vi "Test_NoData_NoneFound.vi"(8 "error in (no error)":errorcluster, 11 "TestCase in":refnum<class "TestCurrentValueTable.lvclass">) -> (0 "error out":errorcluster, 3 "TestCase out":refnum<class "TestCurrentValueTable.lvclass">)   [LabVIEW 2015, in "TestCurrentValueTable.lvclass"]
uses:
  TestCurrentValueTable.lvclass
  <vilib>/addons/_JKI Toolkits/VI Tester/TestCase.llb/TestCase.lvclass
  CurrentValueTable.lvclass
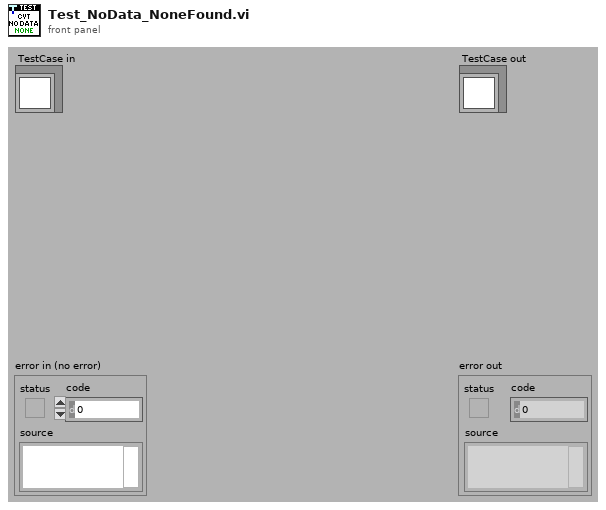
[diagram p1: front panel]
types:
  T1 = typedef "CurrentValueTable.lvlib/CurrentValueTable.lvclass/CurrentValueTable Reference.ctl" = refnum<data-value>
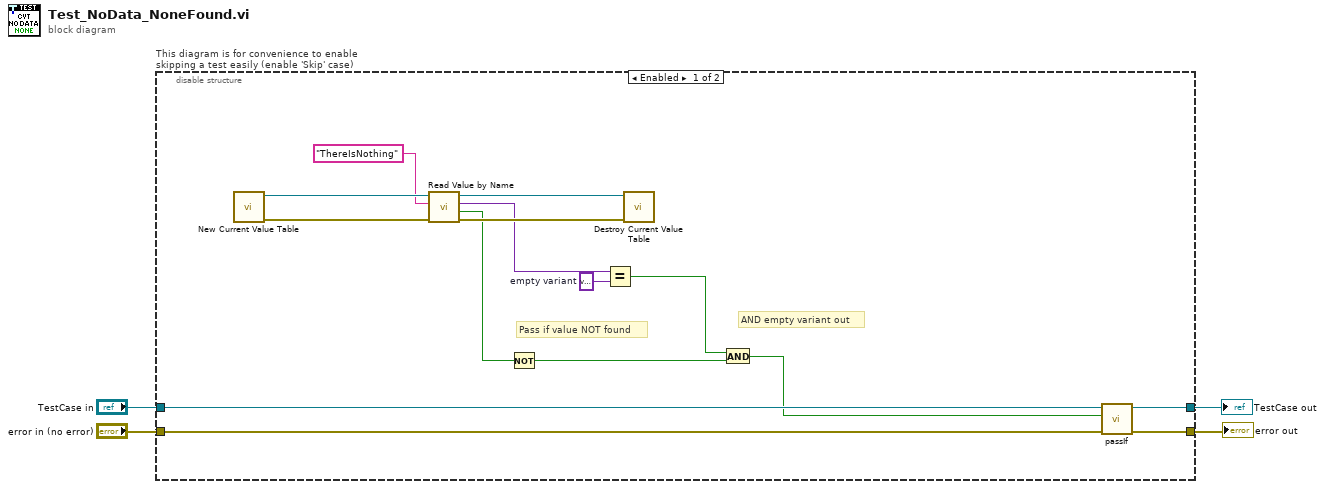
[diagram p0: block diagram]
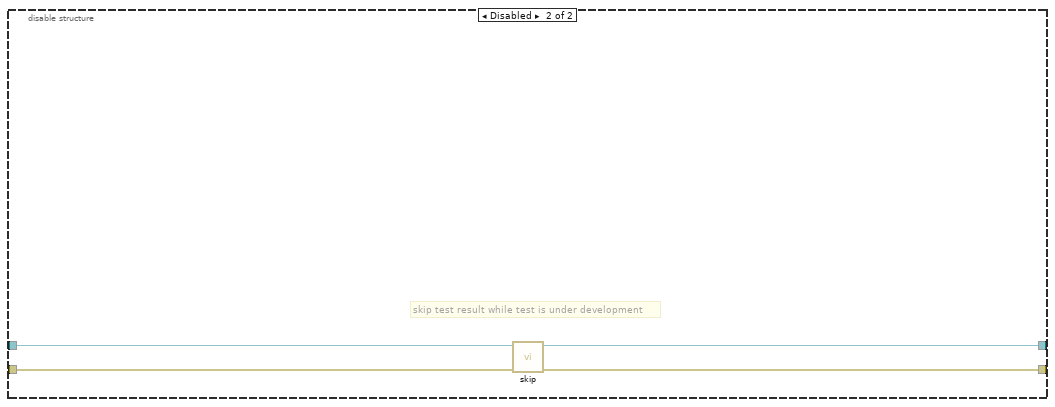
[diagram p2: hidden frame]
diagram:
  n1 = disable-structure "This diagram is for convenience to enable skipping a test easily (enable 'Skip' case)" shown="Enabled" {
    disable-tunnel: "TestCase in" -> [w19 w23]
    disable-tunnel: [w18 w21] -> w1
    disable-tunnel: [w17 w22] -> w3
    disable-tunnel: "error in (no error)" -> [w16 w20]
    frame Enabled {
      w7 = variant  # empty variant
      # "AND empty variant out"
      # "Pass if value NOT found"
      n2 = call "New Current Value Table.vi"() -> ("error out"=w13:errorcluster, "Current Value Table"=w15:T1)  [unwired: 10 in]
      n3 = call "Read Value by Name.vi"("error in (no error)"=w13, "Data Name"="ThereIsNothing", "Current Value Table"=w15) -> ("error out"=w12:errorcluster, "Value Found?"=w10:bool, "Current Value"=w8:variant, "Current Value Table"=w14:T1)  [unwired: 5 in]
      n4 = Not(x=w10) -> (.not. x?=w9:bool)
      n5 = Equal?(x=w8, y=w7) -> (x = y?=w5:bool)
      n6 = call "Destroy Current Value Table.vi"("error in (no error)"=w12, "Current Value Table"=w14) -> ()  [unwired: 9 in, 1 out]
      n7 = And(x=w5, y=w9) -> (x .and. y?=w6:bool)
      n8 = call-dynamic "passIf.vi"("error in (no error)"=w16, "pass"=w6, "TestCase in"=w19) -> ("error out"=w17:errorcluster, "TestCase out"=w18:refnum<class "TestCurrentValueTable.lvclass">)  [unwired: 7 in]
    }
    frame Disabled {
      # "skip test result while test is under development"
      n9 = call <vilib>:"skip.vi"("error in (no error)"=w20, "TestCase in"=w23) -> ("error out"=w22:errorcluster, "TestCase out"=w21:refnum<class "TestCurrentValueTable.lvclass">)  [unwired: 8 in]
    }
  }
  "error out" <- w3
  "TestCase out" <- w1
